vi "Write JSON Config.vi"(6 "Pretty Print?":bool, 8 "error in (no error)":errorcluster, 11 "abs_SharedVar_Bool in":refnum<class "conc_SharedVar_U32.lvclass">) -> (0 "error out":errorcluster, 2 "JSON":string, 3 "abs_SharedVar_Bool out":refnum<class "conc_SharedVar_U32.lvclass">)   [LabVIEW 2021, in "conc_SharedVar_U32.lvclass"]
doc: "LVabs_Shared Variable 1.0.0.2\nTim - TSA\nCopyright (c) 2024, TSA"
uses:
  conc_SharedVar_U32.lvclass
  C:/Program Files (x86)/National Instruments/LabVIEW 2021/vi.lib/TSA/Abstract Data Classes/Abs_Types/Type/Abs_Type.lvclass
  conc_SharedVar_U32.lvclass/conc_SharedVar_U32.ctl
  e6c33842-54ac-4e80-ac0a-ae4d76d05e46.vi
  <vilib>/Utility/LVClass/Get LV Class Name.vi
  <vilib>/JDP Science/JSONtext/Variant to JSON Text.vi
  <vilib>/JDP Science/JSONtext/Set Multiple Object Items.vi
  <vilib>/JDP Science/JSONtext/LVClass Serializer/JSONtext LVClass Serializer.lvclass
  <vilib>/TSA/Abstract Data Classes/Abs_Types/U32 Integer/Abs_U32 Integer.lvclass
  <vilib>/TSA/Abstract Data Classes/Abs_Types/Type/Abs_Type.lvclass
  <vilib>/JDP Science/JSONtext/JSONtext.lvlib
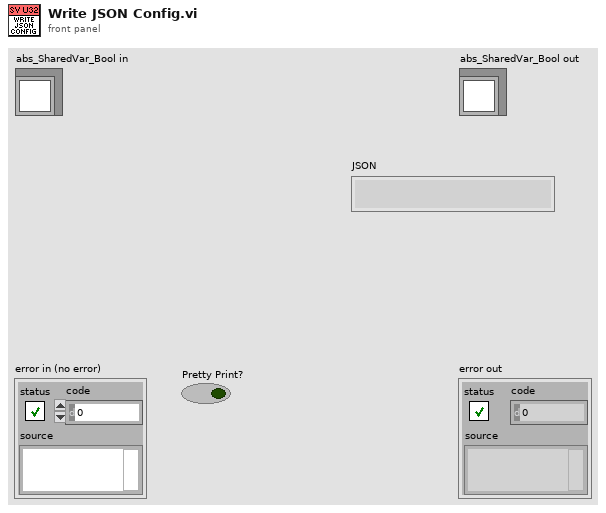
[diagram p1: front panel]
types:
  T1 = cluster{"Shared Variable Refnum":refnum<k21>, "Write Access":enum8{"Allowed", "Required", "None"}, "Read Access":enum8{"Allowed", "Required", "None"}}
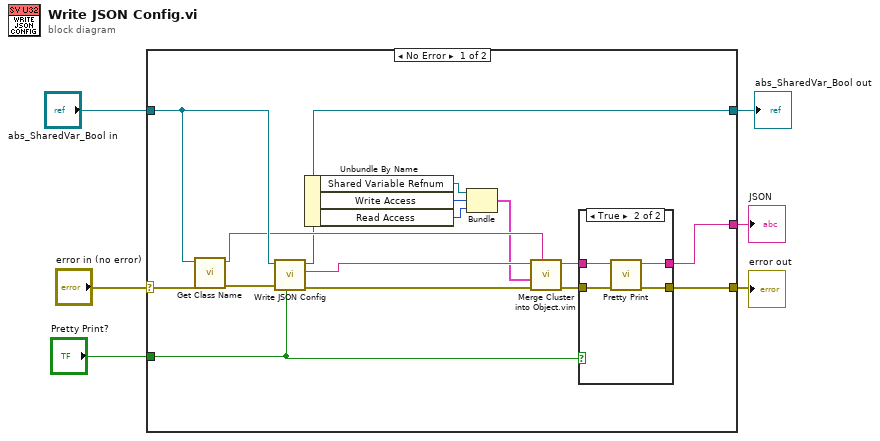
[diagram p0: block diagram]
diagram:
  n1 = case shown="No Error" "error in (no error)" {
    selector: "error in (no error)" -> [w22 w29]
    tunnel: "abs_SharedVar_Bool in" -> [w20 w30]
    tunnel: [w16 w30] -> w4
    tunnel: "Pretty Print?" -> [w9 _]
    tunnel: [w8 w29] -> w2
    tunnel: [w7 _] -> w1
    frame No Error {
      n2 = call <vilib>:"Get Class Name.vi"("error in (no error)"=w22, "Abs_Type in"=w20) -> ("error out"=w21:errorcluster, "class name"=w18:string)  [unwired: 8 in]
      n3 = call-parent "Write JSON Config.vi"("Pretty Print?"=w9, "error in (no error)"=w21, "Abs_Type in"=w20) -> ("error out"=w19:errorcluster, "JSON"=w17:string, "Abs_Type out"=w16:refnum<class "conc_SharedVar_U32.lvclass">)  [unwired: 6 in]
      n4 = Unbundle By Name(w16) -> ("Shared Variable Refnum"=w15:refnum<k21>, "Write Access"=w14:enum8{"Allowed", "Required", "None"}, "Read Access"=w13:enum8{"Allowed", "Required", "None"})
      n5 = Bundle("Shared Variable Refnum"=w15, "Write Access"=w14, "Read Access"=w13) -> (w12:T1)  [unwired: 1 in]
      n6 = call "Merge Cluster into Object.vim"("$Path or Item Name"=w18, "error in (no error)"=w19, "Any Cluster"=w12, "JSON"=w17) -> ("error out"=w11:errorcluster, "<JSON>"=w10:string)  [unwired: 5 in]
      n7 = case shown="True" w9 {
        tunnel: w11 -> [w23 w28]
        tunnel: w10 -> [w24 w27]
        tunnel: [w23 w26] -> w8
        tunnel: [w24 w25] -> w7
        frame False {
        }
        frame True {
          n8 = call <vilib>:"Pretty Print.vi"("error in (no error)"=w28, "JSON"=w27) -> ("error out"=w26:errorcluster, "<JSON>"=w25:string)  [unwired: 7 in, 1 out]
        }
      }
    }
    frame Error {
    }
  }
  "error out" <- w2
  "abs_SharedVar_Bool out" <- w4
  "JSON" <- w1
